vi "ClearTrigger.vi"(8 "Error In":errorcluster, 10 "Line (1-14)":u8=1 min=1 max=14 step=1, 11 "Keithley 2602 In":refnum<visa-resource-name>) -> (0 "Error Out":errorcluster, 3 "Keithley 2602 Out":refnum<visa-resource-name>)   [LabVIEW 2013, in "Keithley-2602.lvlib"]
uses:
  Keithley-2602.lvlib
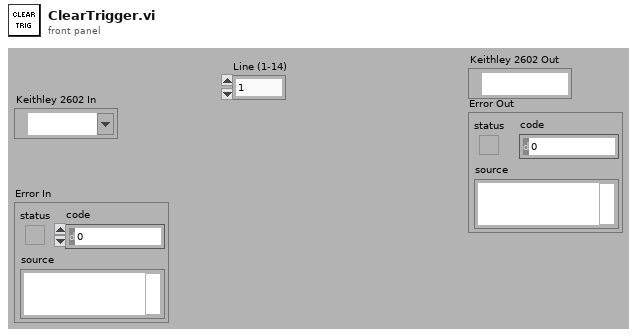
[diagram p1: front panel]
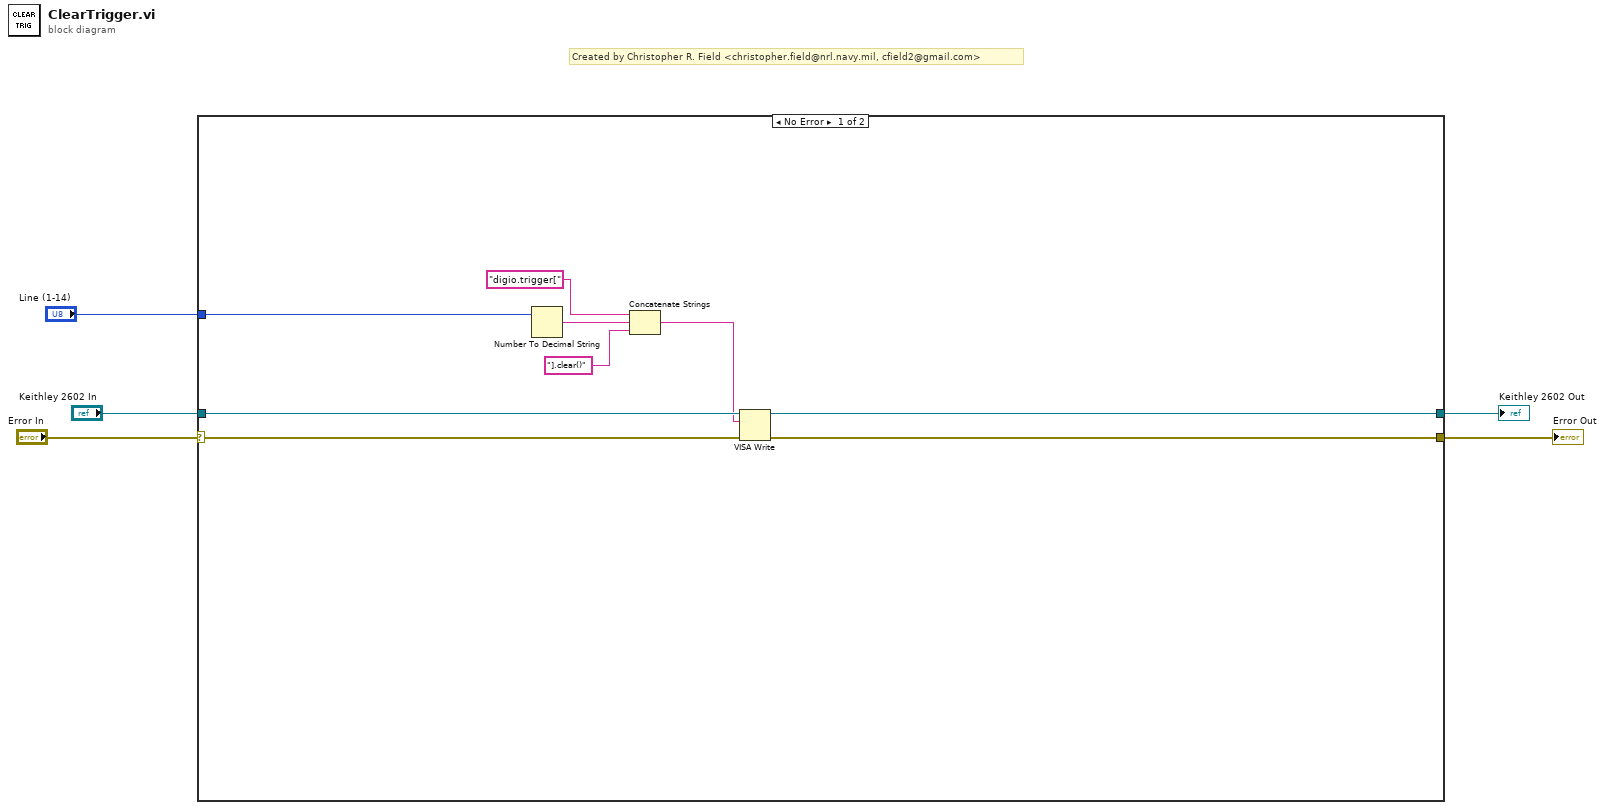
[diagram p0: block diagram]
diagram:
  # "Created by Christopher R. Field <christopher.field@nrl.navy.mil, cfield2@gmail.com>"
  n1 = case shown="No Error" "Error In" {
    selector: "Error In" -> [w6 w15]
    tunnel: "Keithley 2602 In" -> [w14 w16]
    tunnel: [w13 w16] -> w4
    tunnel: [w12 w15] -> w3
    tunnel: "Line (1-14)" -> [w11 _]
    frame No Error {
      n2 = Number To Decimal String(number=w11) -> (decimal integer string=w9:string)  [unwired: 1 in]
      n3 = Concatenate Strings("digio.trigger[", w9, "].clear()") -> (w7:string)
      n4 = VISA Write(VISA resource name=w14, write buffer=w7, error in (no error)=w6) -> (VISA resource name out=w13:refnum<visa-resource-name>, error out=w12:errorcluster)  [unwired: 1 out]
    }
    frame Error {
    }
  }
  "Keithley 2602 Out" <- w4
  "Error Out" <- w3
